vi "ABCtoDQ_noSine_3PhasePowInv.vi"(0 "A":sgl, 1 "cosx":sgl, 2 "sinx":sgl, 5 "B":sgl, 7 "C":sgl, 12 "Resources":T1) -> (4 "direct":sgl, 6 "quadrature":sgl, 10 "alpha":sgl, 15 "beta":sgl)   [LabVIEW 2017]
uses:
  Multiplier/Multiplier.lvclass
  Adder/Adder.lvclass
  Subtractor/Subtractor.lvclass
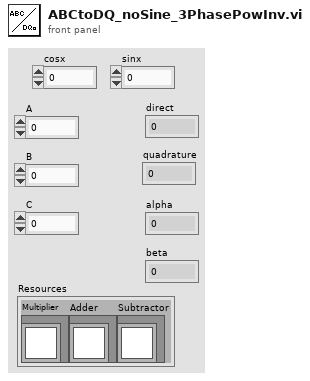
[diagram p1: front panel]
types:
  T1 = cluster{"Multiplier":refnum<class "Multiplier.lvclass">, "Adder":refnum<class "Adder.lvclass">, "Subtractor":refnum<class "Subtractor.lvclass">}
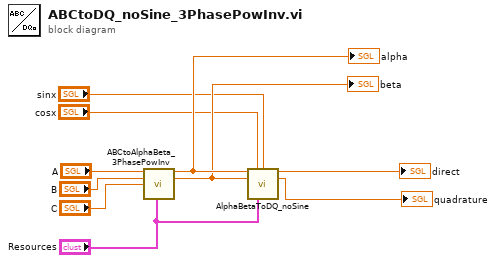
[diagram p0: block diagram]
diagram:
  n1 = call "ABCtoAlphaBeta_3PhasePowInv.vi"("A"="A", "B"="B", "C"="C", "Resources"="Resources") -> ("alpha"=w10:sgl, "beta"=w9:sgl)  [unwired: 10 in]
  "alpha" <- w10
  "beta" <- w9
  n2 = call "AlphaBetaToDQ_noSine.vi"("alpha"=w10, "cosx"="cosx", "sinx"="sinx", "beta"=w9, "Resources"="Resources") -> ("direct"=→"direct":sgl, "quadrature"=→"quadrature":sgl)  [unwired: 9 in]
